vi "K2612 source measure.vi"(0 "VISA Refnum in":refnum<visa-resource-name>, 1 "Sense (2 Wire)":enum32{"2 Wire", "4 Wire", "Calibration"}(ring), 2 "Measure":T2(ring), 5 "Source":enum32{"Current", "Voltage"}(ring), 7 "Channel":T1, 9 "Level (5 V)":dbl, 11 "error in (no error)":errorcluster, 12 "Limit (0.01 A)":dbl, 13 "Measure Count (10)":u32) -> (4 "VISA Refnum out":refnum<visa-resource-name>, 6 "Data Array Out":dbl[](array[numeric]))   [LabVIEW 2018]
uses:
  Program Files/National Instruments/LabVIEW 2023/instr.lib/Keithley 2600 Series old/Keithley 2600 Series.lvlib
  Program Files/National Instruments/LabVIEW 2023/instr.lib/Keithley 2600 Series old/Public/Channel.ctl
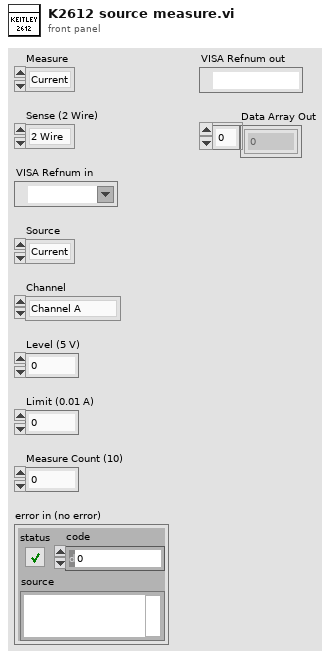
[diagram p1: front panel]
types:
  T1 = typedef "Keithley 2600 Series.lvlib/Channel.ctl" = enum32{"Channel A", "Channel B"}
  T2 = enum32{"Current", "Voltage", "IV", "Resistance", "Power"}
  T3 = enum32{"Normal", "Big Endian", "Little Endian", "Network", "Swapped"}
  T4 = enum32{"ASCII", "Real 32", "Real 64", "Single Precision Real", "Double Precision Real"}
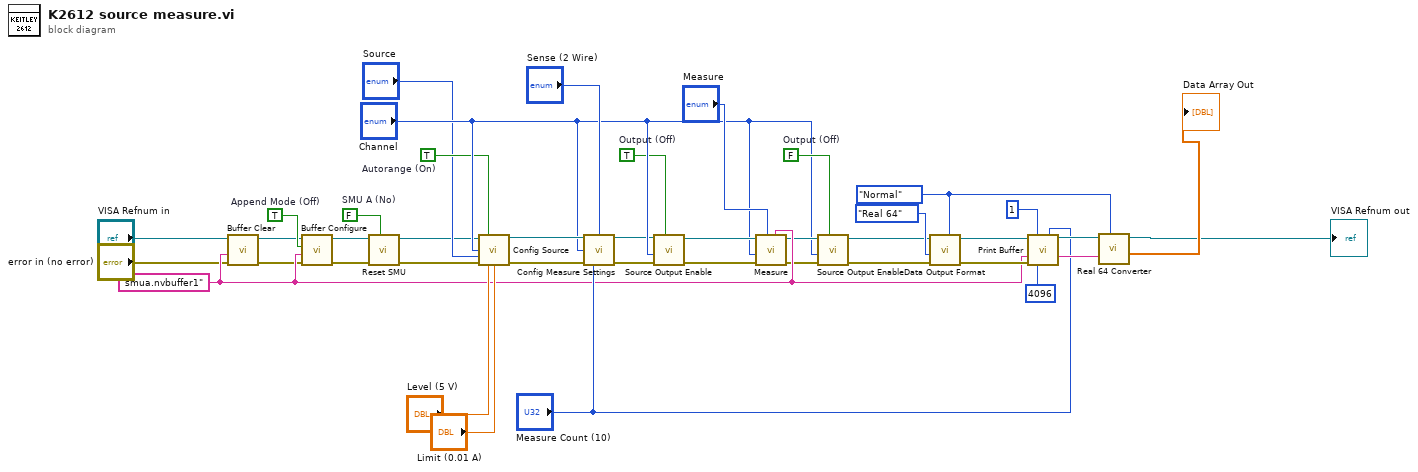
[diagram p0: block diagram]
diagram:
  w33 = T3."Normal" ("Byte Order (Normal)")
  w23 = FALSE  # Output (Off)
  w15 = TRUE  # Output (Off)
  w12 = TRUE  # Autorange (On)
  w8 = FALSE  # SMU A (No)
  w5 = TRUE  # Append Mode (Off)
  w24 = "smua.nvbuffer1" ("Buffer Name")
  n1 = call "Buffer Clear.vi"("error in (no error)"="error in (no error)", "Buffer Name"=w24, "VISA resource name"="VISA Refnum in") -> ("error out"=w4:errorcluster, "VISA resource name out"=w3:refnum<visa-resource-name>)  [unwired: 7 out]
  n2 = call "Buffer Configure.vi"("error in (no error)"=w4, "Buffer Name"=w24, "Append Mode (Off)"=w5, "VISA resource name"=w3) -> ("error out"=w7:errorcluster, "VISA resource name out"=w6:refnum<visa-resource-name>)  [unwired: 3 in, 3 out]
  n3 = call "Reset SMU.vi"("SMU A (No)"=w8, "error in (no error)"=w7, "VISA resource name"=w6) -> ("error out"=w10:errorcluster, "VISA resource name out"=w9:refnum<visa-resource-name>)  [unwired: 2 in, 5 out]
  n4 = call "Config Source.vi"("VISA resource name"=w9, "Autorange (On)"=w12, "Channel (Channel A)"="Channel", "Function (Current)"="Source", "error in"=w10, "Level (0.000)"="Level (5 V)", "Limit (0.1)"="Limit (0.01 A)") -> ("VISA resource name out"=w21:refnum<visa-resource-name>, "error out"=w22:errorcluster)  [unwired: 4 in, 3 out]
  n5 = call "Config Measure Settings.vi"("VISA resource name"=w21, "Sense (2 Wire)"="Sense (2 Wire)", "Channel (Channel A)"="Channel", "error in"=w22, "Measure Count (1)"="Measure Count (10)") -> ("VISA resource name out"=w13:refnum<visa-resource-name>, "error out"=w14:errorcluster)  [unwired: 5 in, 4 out]
  n6 = call "Source Output Enable.vi"("Output (Off)"=w15, "error in (no error)"=w14, "Channel (Channel A)"="Channel", "VISA resource name"=w13) -> ("error out"=w17:errorcluster, "VISA resource name out"=w18:refnum<visa-resource-name>)  [unwired: 1 in, 5 out]
  n7 = call "Measure.vi"("Buffer 1"=w24, "Function (Current)"="Measure", "error in (no error)"=w17, "Channel (Channel A)"="Channel", "VISA resource name"=w18) -> ("error out"=w20:errorcluster, "VISA resource name out"=w19:refnum<visa-resource-name>)  [unwired: 2 in, 3 out]
  n8 = call "Source Output Enable.vi"("Output (Off)"=w23, "error in (no error)"=w20, "Channel (Channel A)"="Channel", "VISA resource name"=w19) -> ("error out"=w29:errorcluster, "VISA resource name out"=w28:refnum<visa-resource-name>)  [unwired: 1 in, 5 out]
  n9 = call "Data Output Format.vi"("Byte Order (Normal)"=w33, "error in (no error)"=w29, "Data Format (ASCII)"=T4."Real 64", "VISA resource name"=w28) -> ("error out"=w31:errorcluster, "VISA resource name out"=w32:refnum<visa-resource-name>)  [unwired: 2 in, 4 out]
  n10 = call "Print Buffer.vi"("VISA resource name"=w32, "Start Index (1)"=u32 1, "End Index (1)"="Measure Count (10)", "Buffer Name(s)"=w24, "error in (no error)"=w31, "Byte Count (1024)"=u32 4096) -> ("VISA resource name out"=→"VISA Refnum out":refnum<visa-resource-name>, "Buffer Data"=w36:string)  [unwired: 1 in, 7 out]
  n11 = call "Real 64 Converter.vi"("Byte Order (Normal)"=w33, "Data In"=w36) -> ("Data Array Out"=→"Data Array Out":dbl[])  [unwired: 9 out]
